vi "HoloPy_Find_Features.vi"(8 "error in (no error)":errorcluster, 9 "imageNumber":i32, 10 "Threshold":dbl, 11 "Refnum in":refnum<k35>) -> (0 "error out":errorcluster, 2 "FEATURES(µm)":sgl[][](array[numeric]), 3 "Refnum out":refnum<k35>)   [LabVIEW 2023, in "holoPyTracks.lvlib"]
uses:
  holoPyTracks.lvlib
panel:
  # "Python Node in holoPY.lvlib:HoloPy_Find_Features.vi->holoPY.lvlib:HoloPy_Example.vi<APPEND>\n\nPython returned the following error: Type mismatch while marshaling Python array. Expected type: float, received: void."
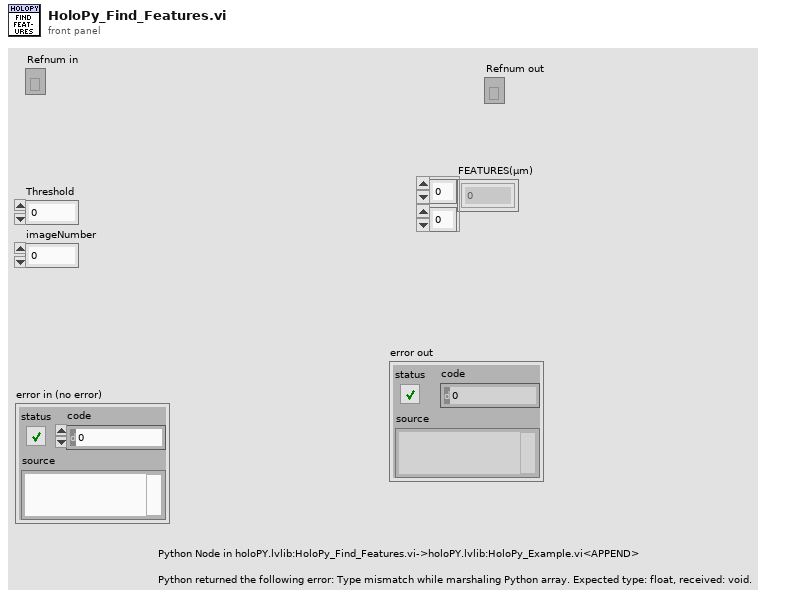
[diagram p1: front panel]
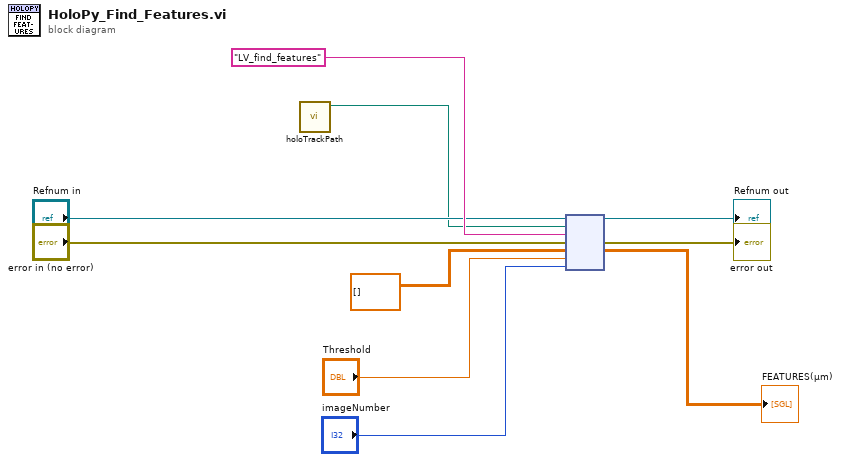
[diagram p0: block diagram]
diagram:
  n1 = call "holoTrackPath.vi"() -> ("appended path"=w1:path)  [unwired: 11 in]
  n2 = node("Refnum in", w1, "LV_find_features" ("function name"), "error in (no error)", sgl[][] [], "Threshold", "imageNumber") -> (→"Refnum out":refnum<k35>, →"error out":errorcluster, →"FEATURES(µm)":sgl[][])  [unwired: 2 in, 2 out]
